vi "set_example.vi"() -> ()   [LabVIEW 2021]
panel:
  out "Array":i32[](array[numeric])
  out "set in":set{i32}(c389)
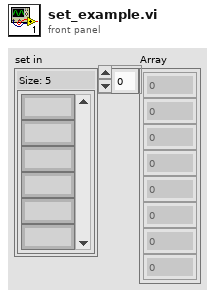
[diagram p1: front panel]
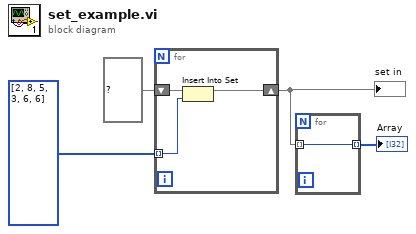
[diagram p0: block diagram]
diagram:
  n1 = for {
    shift-right: [w5] -> w2
    shift-left: set{i32} {} ("set in") -> [w7]
    tunnel: i32[] [2, 8, 5, 3, 6, 6] -> [w6] mode=indexing
    n2 = Insert Into Set(10:w6, 11:w7) -> (3:w5:set{i32})  [unwired: 1 out]
  }
  "set in" <- w2
  n3 = for {
    tunnel: w2 -> [w8] mode=indexing
    tunnel: [w8] -> w1 mode=indexing
  }
  "Array" <- w1
